vi "Outputs.vi"(8 "error in (no error)":errorcluster, 11 "State in":T1={"State"=enum."Idle", "Start Time"=timestamp(0 s since 1904-01-01), "Configuration"={"Cycle Period"=0.0, "Manual Entry"=0.0, "Output Device"=enum."Ismatec ISM 831C", "Ismatech"={"VISA resource name"="", "Simulated?"=FALSE, "Pump Number"=1.0, "Reverse?"=FALSE}, "Ismatech 3 Channel Settings"={"VISA resource name"="", "Pump Number"=1, "Channel Number"=0, "Simulated?"=TRUE, "Reverse?"=FALSE}, "Masterflex"={"VISA resource name"="", "Simulated?"=FALSE, "Pump Number"=1.0, "Reverse?"=FALSE}, "VICI Settings"={"VISA resource name"="", "Pump ID"="", "Pump Head Vol"=0.0, "Reverse?"=FALSE, "Simulated?"=FALSE}, "Tacmina Settings"={"Analog DAQ Task"="", "Digital DAQ Task"=""}, "KNF SIMDOS Settings"={"VISA resource name"="", "Simulated?"=TRUE}, "ASIA Pump C"={"ASIA Pump #"=0, "channel"=0, "Simulated"=FALSE}, "FLOM Settings"={"VISA resource name"="", "Simulated?"=TRUE, "Pump Number"=0.0}, "SSI PR/LD Settings"={"VISA resource name"="", "Simulated?"=FALSE}, "SSI P40 Settings"={"VISA resource name"="", "Simulated?"=FALSE}, "Masterflex 75211 Settings"={"Analog DAQ Task"="", "Digital DAQ Task"=""}, "Pump Calibration File"=path "", "Calibration Slope"=0.0, "Calibration Y Intercept"=0.0, "Pump Cal Enum"=0, "Reset Totalizer"=FALSE}, "Current Time"=timestamp(0 s since 1904-01-01), "First Iteration"=FALSE, "Data"={"Pump Speed"=0.0, "Pump Pressure"=0.0, "Pump Flow"=0.0, "Totalized"=0.0}, "Process Name"="", "Pump On?"=enum."Off", "Output Error"=FALSE, "Log Started"=FALSE, "Overpressure Alarming"=FALSE} {"Configuration"."Ismatech 3 Channel Settings"."Channel Number" min=0 max=3; "Configuration"."Ismatech 3 Channel Settings"."Pump Number" min=1; "Configuration"."ASIA Pump C"."channel" min=0 max=1 step=1; "Configuration"."Masterflex"."Pump Number" min=1.0 max=20.0 step=1.0; "Configuration"."Ismatech"."Pump Number" min=1.0 max=20.0 step=1.0}) -> (0 "error out":errorcluster, 3 "State out":T1={"State"=enum."Idle", "Start Time"=timestamp(0 s since 1904-01-01), "Configuration"={"Cycle Period"=0.0, "Manual Entry"=0.0, "Output Device"=enum."Ismatec ISM 831C", "Ismatech"={"VISA resource name"="", "Simulated?"=FALSE, "Pump Number"=1.0, "Reverse?"=FALSE}, "Ismatech 3 Channel Settings"={"VISA resource name"="", "Pump Number"=1, "Channel Number"=0, "Simulated?"=TRUE, "Reverse?"=FALSE}, "Masterflex"={"VISA resource name"="", "Simulated?"=FALSE, "Pump Number"=1.0, "Reverse?"=FALSE}, "VICI Settings"={"VISA resource name"="", "Pump ID"="", "Pump Head Vol"=0.0, "Reverse?"=FALSE, "Simulated?"=FALSE}, "Tacmina Settings"={"Analog DAQ Task"="", "Digital DAQ Task"=""}, "KNF SIMDOS Settings"={"VISA resource name"="", "Simulated?"=TRUE}, "ASIA Pump C"={"ASIA Pump #"=0, "channel"=0, "Simulated"=FALSE}, "FLOM Settings"={"VISA resource name"="", "Simulated?"=TRUE, "Pump Number"=0.0}, "SSI PR/LD Settings"={"VISA resource name"="", "Simulated?"=FALSE}, "SSI P40 Settings"={"VISA resource name"="", "Simulated?"=FALSE}, "Masterflex 75211 Settings"={"Analog DAQ Task"="", "Digital DAQ Task"=""}, "Pump Calibration File"=path "", "Calibration Slope"=0.0, "Calibration Y Intercept"=0.0, "Pump Cal Enum"=0, "Reset Totalizer"=FALSE}, "Current Time"=timestamp(0 s since 1904-01-01), "First Iteration"=FALSE, "Data"={"Pump Speed"=0.0, "Pump Pressure"=0.0, "Pump Flow"=0.0, "Totalized"=0.0}, "Process Name"="", "Pump On?"=enum."Off", "Output Error"=FALSE, "Log Started"=FALSE, "Overpressure Alarming"=FALSE} {"Configuration"."Ismatech 3 Channel Settings"."Channel Number" min=0 max=3; "Configuration"."Ismatech 3 Channel Settings"."Pump Number" min=1; "Configuration"."ASIA Pump C"."channel" min=0 max=1 step=1; "Configuration"."Masterflex"."Pump Number" min=1.0 max=20.0 step=1.0; "Configuration"."Ismatech"."Pump Number" min=1.0 max=20.0 step=1.0})   [LabVIEW 2018, in "Pump Module.lvlib" / "Pump Module Engine.lvlib"]
uses:
  Pump Module Engine.lvlib
  State Cluster.ctl
  State Enum.ctl
  Pump Module Settings Cluster.ctl
  Measure Instrument/PID 2 Output Enum.ctl
  Ismatec ISM 831C/Controls/Ismatech ISM831C Settings Cluster.ctl
  Ismatec 78001/Ismatec 4083.ctl
  Masterflex 7550-30/Controls/Settings Cluster.ctl
  VICI M50 Party Mode/Settings Cluster.ctl
  Tacmina QI/Tacmina QI DAQ Setting.ctl
  KNF Pump/Settings Cluster plus SIMDOS.ctl
  ASIA Pump/Pump Settings.ctl
  FLOM Pump/Settings Cluster.ctl
  SSI PR Class/SSI PR or LD Settings Cluster.ctl
  Masterflex 75211/Masterflex 75211 DAQ Setting.ctl
  Pump Settings Cluster.ctl
  Tag VIs/Tag FGV Operation Enum.ctl
  Shared Variables/Dynamic Shared Variables.lvlib
  Masterflex 7550-30/Masterflex 7550-30.lvlib
  Ismatec ISM 831C/Ismatec ISM 831C.lvlib
  VICI M50 Party Mode/VICI M6 M50 Party Mode.lvlib
  Tacmina QI/Tacmina QI.lvlib
  KNF Pump/KNF SIMDOS.lvlib
  ASIA Pump.lvlib
  FLOM Pump/FLOM Pump.lvlib
  SSI PR Class/SSI PR or LD Pump.lvlib
  Pump Module.lvlib
  Masterflex 75211/Masterflex 75211.lvlib
  Ismatec 78001/Ismatec 4308.lvlib
panel:
  # "Output Instruments"
  # "Output Instruments"
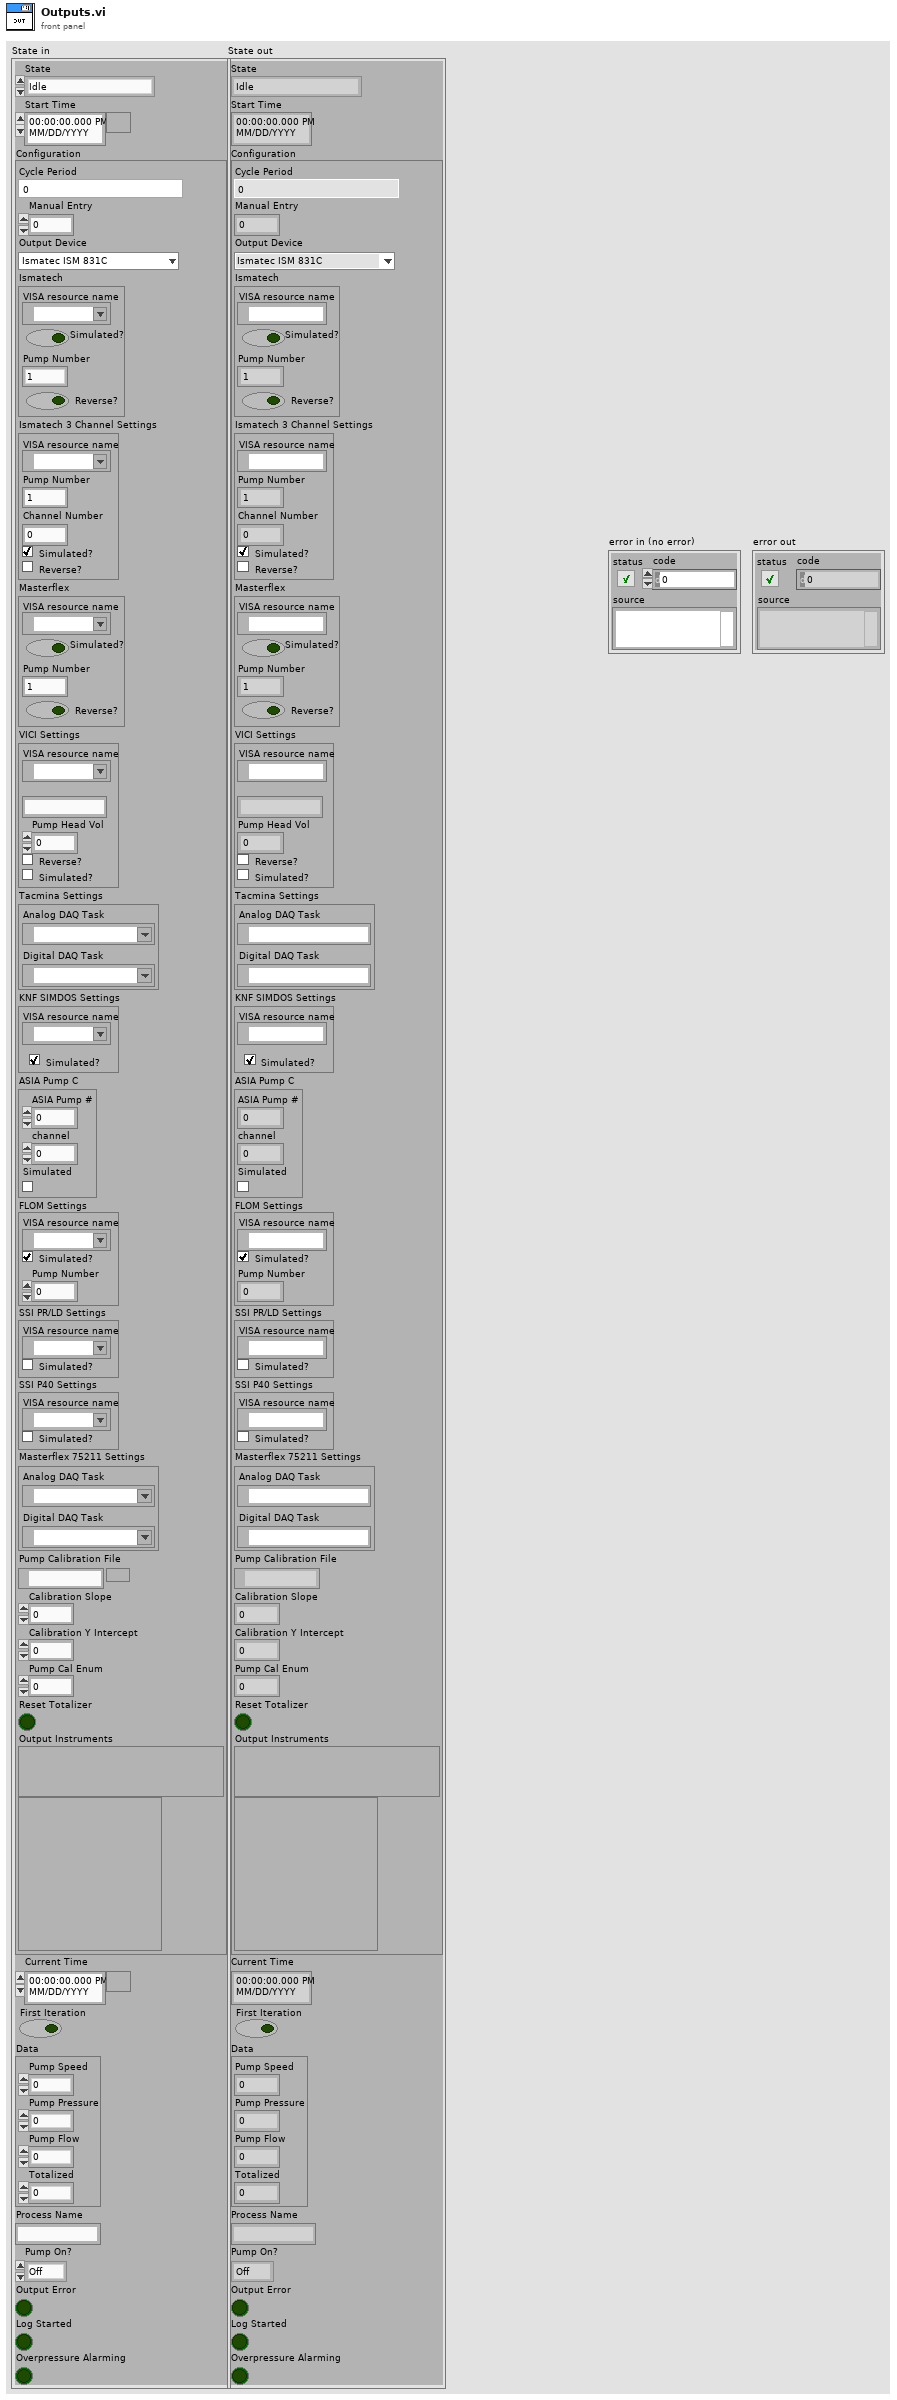
[diagram p1: front panel]
types:
  T1 = typedef "Pump Module.lvlib/Pump Module Engine.lvlib/State Cluster.ctl" = cluster{"State":T2, "Start Time":timestamp, "Configuration":T3, "Current Time":timestamp, "First Iteration":bool, "Data":cluster{"Pump Speed":dbl, "Pump Pressure":dbl, "Pump Flow":dbl, "Totalized":dbl}, "Process Name":string, "Pump On?":enum16{"Off", "On", "Not Initialized"}, "Output Error":bool, "Log Started":bool, "Overpressure Alarming":bool}
  T2 = typedef "Pump Module.lvlib/Pump Module Engine.lvlib/State Enum.ctl" = enum16{"Measuring", "Idle", "Paused"}
  T3 = typedef "Pump Module.lvlib/Pump Module Settings Cluster.ctl" = cluster{"Cycle Period":dbl, "Manual Entry":dbl, "Output Device":T4, "Ismatech":T5, "Ismatech 3 Channel Settings":T6, "Masterflex":T7, "VICI Settings":T8, "Tacmina Settings":T9, "KNF SIMDOS Settings":T10, "ASIA Pump C":T11, "FLOM Settings":T12, "SSI PR/LD Settings":T13, "SSI P40 Settings":T13, "Masterflex 75211 Settings":T14, "Pump Calibration File":path, "Calibration Slope":dbl, "Calibration Y Intercept":dbl, "Pump Cal Enum":u16, "Reset Totalizer":bool}
  T4 = typedef "PID 2 Output Enum.ctl" = enum16{"Default", "Ismatec ISM 4308", "Ismatec ISM 831C", "Masterflex 7550-30", "VICI M6", "VICI M50", "Tacmina QI", "KNF SIMDOS", "ASIA Type C", "FLOM UI-22-11", "SSI PR/LD", "SSI P40", "Masterflex 75211-70"}
  T5 = typedef "Ismatec ISM 831C.lvlib/Ismatech ISM831C Settings Cluster.ctl" = cluster{"VISA resource name":refnum<visa-resource-name>, "Simulated?":bool, "Pump Number":dbl, "Reverse?":bool}
  T6 = typedef "Ismatec 4308.lvlib/Ismatec 4083.ctl" = cluster{"VISA resource name":refnum<visa-resource-name>, "Pump Number":i16, "Channel Number":i16, "Simulated?":bool, "Reverse?":bool}
  T7 = typedef "Masterflex 7550-30.lvlib/Settings Cluster.ctl" = cluster{"VISA resource name":refnum<visa-resource-name>, "Simulated?":bool, "Pump Number":dbl, "Reverse?":bool}
  T8 = typedef "VICI M6 M50 Party Mode.lvlib/Settings Cluster.ctl" = cluster{"VISA resource name":refnum<visa-resource-name>, "Pump ID":string, "Pump Head Vol":dbl, "Reverse?":bool, "Simulated?":bool}
  T9 = typedef "Tacmina QI.lvlib/Tacmina QI DAQ Setting.ctl" = cluster{"Analog DAQ Task":refnum<k21>, "Digital DAQ Task":refnum<k21>}
  T10 = typedef "KNF SIMDOS.lvlib/Settings Cluster plus SIMDOS.ctl" = cluster{"VISA resource name":refnum<visa-resource-name>, "Simulated?":bool}
  T11 = typedef "ASIA Pump.lvlib/Pump Settings.ctl" = cluster{"ASIA Pump #":i32, "channel":i32, "Simulated":bool}
  T12 = typedef "FLOM Pump.lvlib/Settings Cluster.ctl" = cluster{"VISA resource name":refnum<visa-resource-name>, "Simulated?":bool, "Pump Number":dbl}
  T13 = typedef "SSI PR or LD Pump.lvlib/SSI PR or LD Settings Cluster.ctl" = cluster{"VISA resource name":refnum<visa-resource-name>, "Simulated?":bool}
  T14 = typedef "Masterflex 75211.lvlib/Masterflex 75211 DAQ Setting.ctl" = cluster{"Analog DAQ Task":refnum<k21>, "Digital DAQ Task":refnum<k21>}
  T15 = typedef "Tag FGV Operation Enum.ctl" = enum16{"Init", "Set Notification Queue", "Create Tag", "Commit", "Write Tag (Numeric)", "Write Tag (Boolean)", "Read All Tags", "Read One Tag", "Delete Tag Category", "Set Alarm Parameters (Numeric)", "Set Alarm Parameters (Boolean)", "Enable All Alarms", "Disable All Alarms", "Delete All Tags", "Read Alarms", "Ack Alarm", "Read Alarm Parameters (Numeric)", "Read Alarm Parameters (Boolean)"}
  T16 = typedef "Pump Module.lvlib/Pump Settings Cluster.ctl" = cluster{"Output Device":T4, "Masterflex":T7, "Ismatech":T5, "Ismatech 3 Channel Settings":T6, "VICI Settings":T8, "Tacmina Settings":T9, "KNF SIMDOS Settings":T10, "ASIA Pump C":T11, "FLOM Settings":T12, "SSI PR/LD Settings":T13, "SSI P40 Settings":T13, "Masterflex 75211 Settings":T14}
  T17 = typedef "Pump Module.lvlib/Pump Module Tag Names Cluster.ctl" = cluster{"Pump Speed":string, "Totalized g Tag":string, "Pump Flow":string, "Pump Pressure":string, "Output Device Tag":string, "Overpressure Tag":string, "Identifier Tag":string}
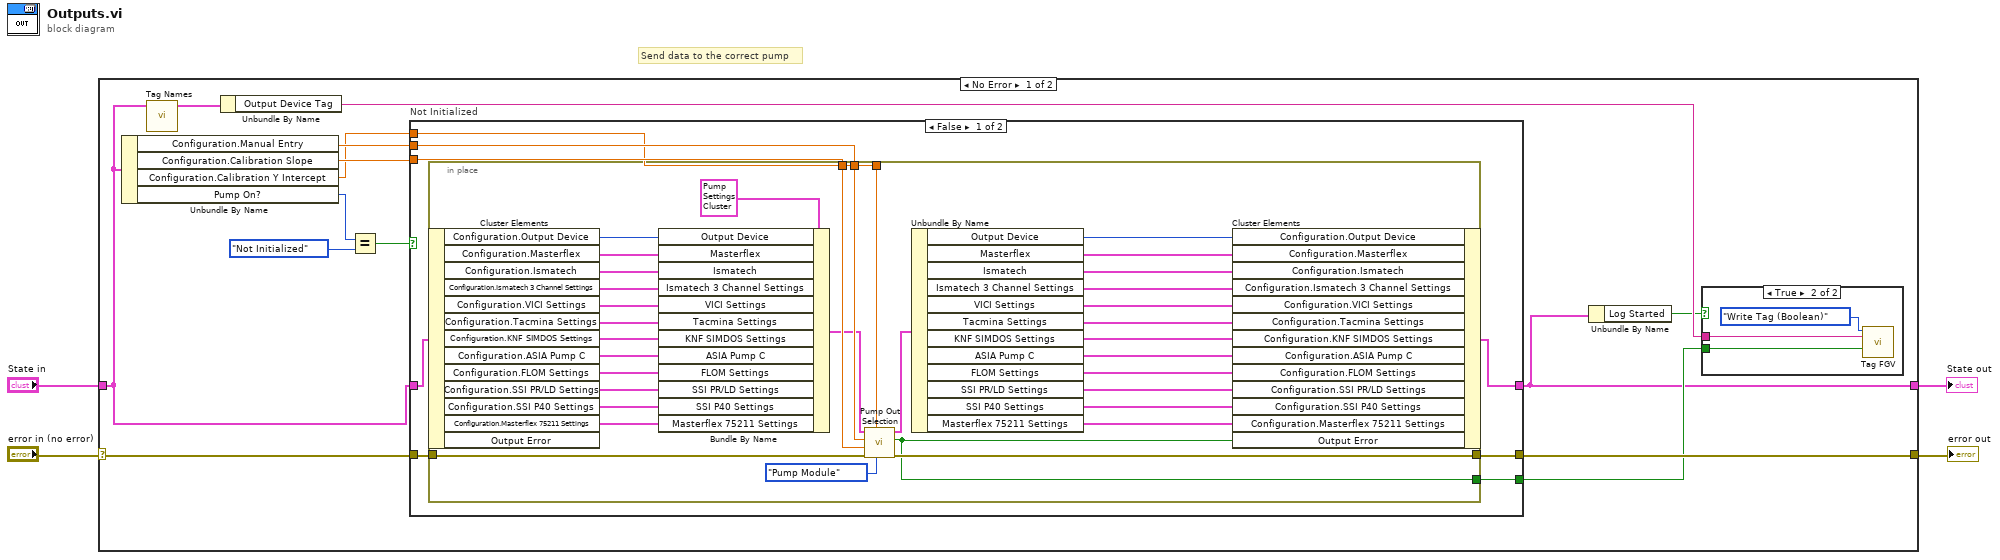
[diagram p0: block diagram]
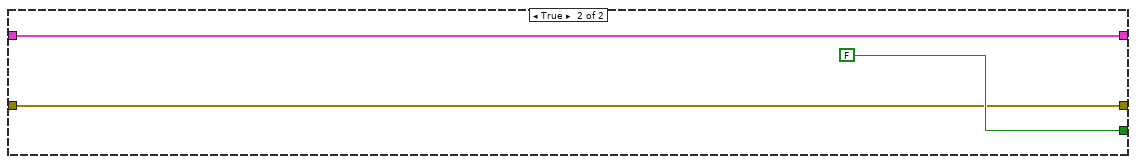
[diagram p3: hidden frame]
diagram:
  # "Send data to the correct pump"
  n1 = case shown="No Error" "error in (no error)" {
    selector: "error in (no error)" -> [w18 w68]
    tunnel: [w16 w68] -> w3
    tunnel: "State in" -> [w9 w67]
    tunnel: [w8 w67] -> w1
    frame No Error {
      n2 = Unbundle By Name(w9) -> ("Configuration.Manual Entry"=w10:dbl, "Configuration.Calibration Slope"=w11:dbl, "Configuration.Calibration Y Intercept"=w7:dbl, "Pump On?"=w5:enum16{"Off", "On", "Not Initialized"})
      n3 = call "Tag Names.vi"("State In"=w9) -> ("Pump Module Tag Names"=w17:T17)  [unwired: 8 in, 2 out]
      n4 = Unbundle By Name(w17) -> ("Output Device Tag"=w15:string)
      n5 = Equal?(x=w5, y=enum16{"Off", "On", "Not Initialized"}."Not Initialized" ("x")) -> (x = y?=w13:bool)
      n6 = case "Not Initialized" shown="False" w13 {
        tunnel: w11 -> [w29 _]
        tunnel: w18 -> [w28 w65]
        tunnel: [w27 w65] -> w16
        tunnel: [w25 FALSE ("Connection Error")] -> w14
        tunnel: w10 -> [w26 _]
        tunnel: w9 -> [w23 w64]
        tunnel: [w22 w64] -> w8
        tunnel: w7 -> [w24 _]
        frame False {
          n7 = in-place {
            in-place-border: w29 -> [w63]
            in-place-border: w28 -> [w62]
            in-place-border: [w61] -> w27
            in-place-border: w26 -> [w60]
            in-place-border: [w36] -> w25
            in-place-border: w24 -> [w55]
            n8 = in-place-cluster #1(w23) -> ("Configuration.Output Device"=w54:T4, "Configuration.Masterflex"=w53:T7, "Configuration.Ismatech"=w52:T5, "Configuration.Ismatech 3 Channel Settings"=w31:T6, "Configuration.VICI Settings"=w51:T8, "Configuration.Tacmina Settings"=w50:T9, "Configuration.KNF SIMDOS Settings"=w49:T10, "Configuration.ASIA Pump C"=w48:T11, "Configuration.FLOM Settings"=w47:T12, "Configuration.SSI PR/LD Settings"=w46:T13, "Configuration.SSI P40 Settings"=w32:T13, "Configuration.Masterflex 75211 Settings"=w35:T14)  [unwired: 1 out]
            n9 = Bundle By Name(cluster=T16 {"Output Device"=enum."Default", "Masterflex"={"VISA resource name"="", "Simulated?"=FALSE, "Pump Number"=0.0, "Reverse?"=FALSE}, "Ismatech"={"VISA resource name"="", "Simulated?"=FALSE, "Pump Number"=0.0, "Reverse?"=FALSE}, "Ismatech 3 Channel Settings"={"VISA resource name"="", "Pump Number"=1, "Channel Number"=0, "Simulated?"=TRUE, "Reverse?"=FALSE}, "VICI Settings"={"VISA resource name"="", "Pump ID"="", "Pump Head Vol"=0.0, "Reverse?"=FALSE, "Simulated?"=FALSE}, "Tacmina Settings"={"Analog DAQ Task"="", "Digital DAQ Task"=""}, "KNF SIMDOS Settings"={"VISA resource name"="", "Simulated?"=FALSE}, "ASIA Pump C"={"ASIA Pump #"=0, "channel"=0, "Simulated"=FALSE}, "FLOM Settings"={"VISA resource name"="", "Simulated?"=FALSE, "Pump Number"=0.0}, "SSI PR/LD Settings"={"VISA resource name"="", "Simulated?"=FALSE}, "SSI P40 Settings"={"VISA resource name"="", "Simulated?"=FALSE}, "Masterflex 75211 Settings"={"Analog DAQ Task"="", "Digital DAQ Task"=""}} ("Pump Settings Out"), "Output Device"=w54, "Masterflex"=w53, "Ismatech"=w52, "Ismatech 3 Channel Settings"=w31, "VICI Settings"=w51, "Tacmina Settings"=w50, "KNF SIMDOS Settings"=w49, "ASIA Pump C"=w48, "FLOM Settings"=w47, "SSI PR/LD Settings"=w46, "SSI P40 Settings"=w32, "Masterflex 75211 Settings"=w35) -> (w57:T16)
            n10 = call "Pump Out Selection.vi"("Module Type"=enum16{"Feed Module", "Pump Module"}."Pump Module", "Calibration Y Intercept"=w55, "error in (no error)"=w62, "Calibration Slope"=w63, "Speed"=w60, "Pump Settings In"=w57) -> ("error out"=w61:errorcluster, "Connection Error"=w36:bool, "Pump Settings Out"=w56:T16)  [unwired: 3 in]
            n11 = Unbundle By Name(w56) -> ("Output Device"=w45:T4, "Masterflex"=w44:T7, "Ismatech"=w43:T5, "Ismatech 3 Channel Settings"=w30:T6, "VICI Settings"=w42:T8, "Tacmina Settings"=w41:T9, "KNF SIMDOS Settings"=w40:T10, "ASIA Pump C"=w39:T11, "FLOM Settings"=w38:T12, "SSI PR/LD Settings"=w37:T13, "SSI P40 Settings"=w33:T13, "Masterflex 75211 Settings"=w34:T14)
            n12 = in-place-cluster #1("Configuration.Output Device"=w45, "Configuration.Masterflex"=w44, "Configuration.Ismatech"=w43, "Configuration.Ismatech 3 Channel Settings"=w30, "Configuration.VICI Settings"=w42, "Configuration.Tacmina Settings"=w41, "Configuration.KNF SIMDOS Settings"=w40, "Configuration.ASIA Pump C"=w39, "Configuration.FLOM Settings"=w38, "Configuration.SSI PR/LD Settings"=w37, "Configuration.SSI P40 Settings"=w33, "Configuration.Masterflex 75211 Settings"=w34, "Output Error"=w36) -> (w22:T1)
          }
        }
        frame True {
        }
      }
      n13 = Unbundle By Name(w8) -> ("Log Started"=w12:bool)
      n14 = case shown="True" w12 {
        tunnel: w15 -> [_ w21]
        tunnel: w14 -> [_ w20]
        frame False {
        }
        frame True {
          n15 = call "Tag FGV.vi"("Operation"=Tag_FGV_Operation_Enum."Write Tag (Boolean)", "Tag Name"=w21, "Data"=w20) -> ()  [unwired: 5 in, 8 out]
        }
      }
    }
    frame Error {
    }
  }
  "error out" <- w3
  "State out" <- w1
